vi "Change Detect.vi"(4 "Value":variant) -> (1 "Changed?":bool)   [LabVIEW 2016]
doc: "Report if input has changed since previous call. Always true on first call."
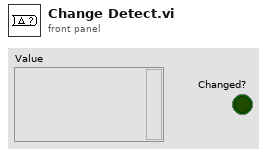
[diagram p1: front panel]
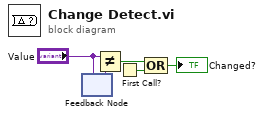
[diagram p0: block diagram]
diagram:
  n1 = feedback-in #1("Value") -> ()
  n2 = feedback #1() -> (w3:variant)  [unwired: 1 in]
  n3 = Not Equal?(x="Value", y=w3) -> (x != y?=w1:bool)
  n4 = First Call?() -> (First Call?: T/F=w5:bool)
  n5 = Compound Arithmetic op=OR(w1, w5) -> (→"Changed?":bool)
